vi "cupFinderv5.vi"(11 "image\n in":T1(plugin-control)) -> (0 "WORK FOR GODS SAKE 2":T1(plugin-control), 1 "X-Out":dbl, 2 "CupPosition":T1(plugin-control), 3 "Refnum out":T1(plugin-control), 4 "Y-Out":dbl, 5 "ImgToCrop":T1(plugin-control))   [LabVIEW 2017]
uses:
  <vilib>/vision/NI_Vision_Development_Module.lvlib
panel:
  out "ROI Descriptor":T2 {"Contours"."Type" items=["No Selection", "Point", "Line", "Rectangle", "Oval", "Polygon", "Freehand Region", "Annulus", "Unused2", "Unused3", "Broken Line", "Freehand Line", "Rotated Rectangle"]}
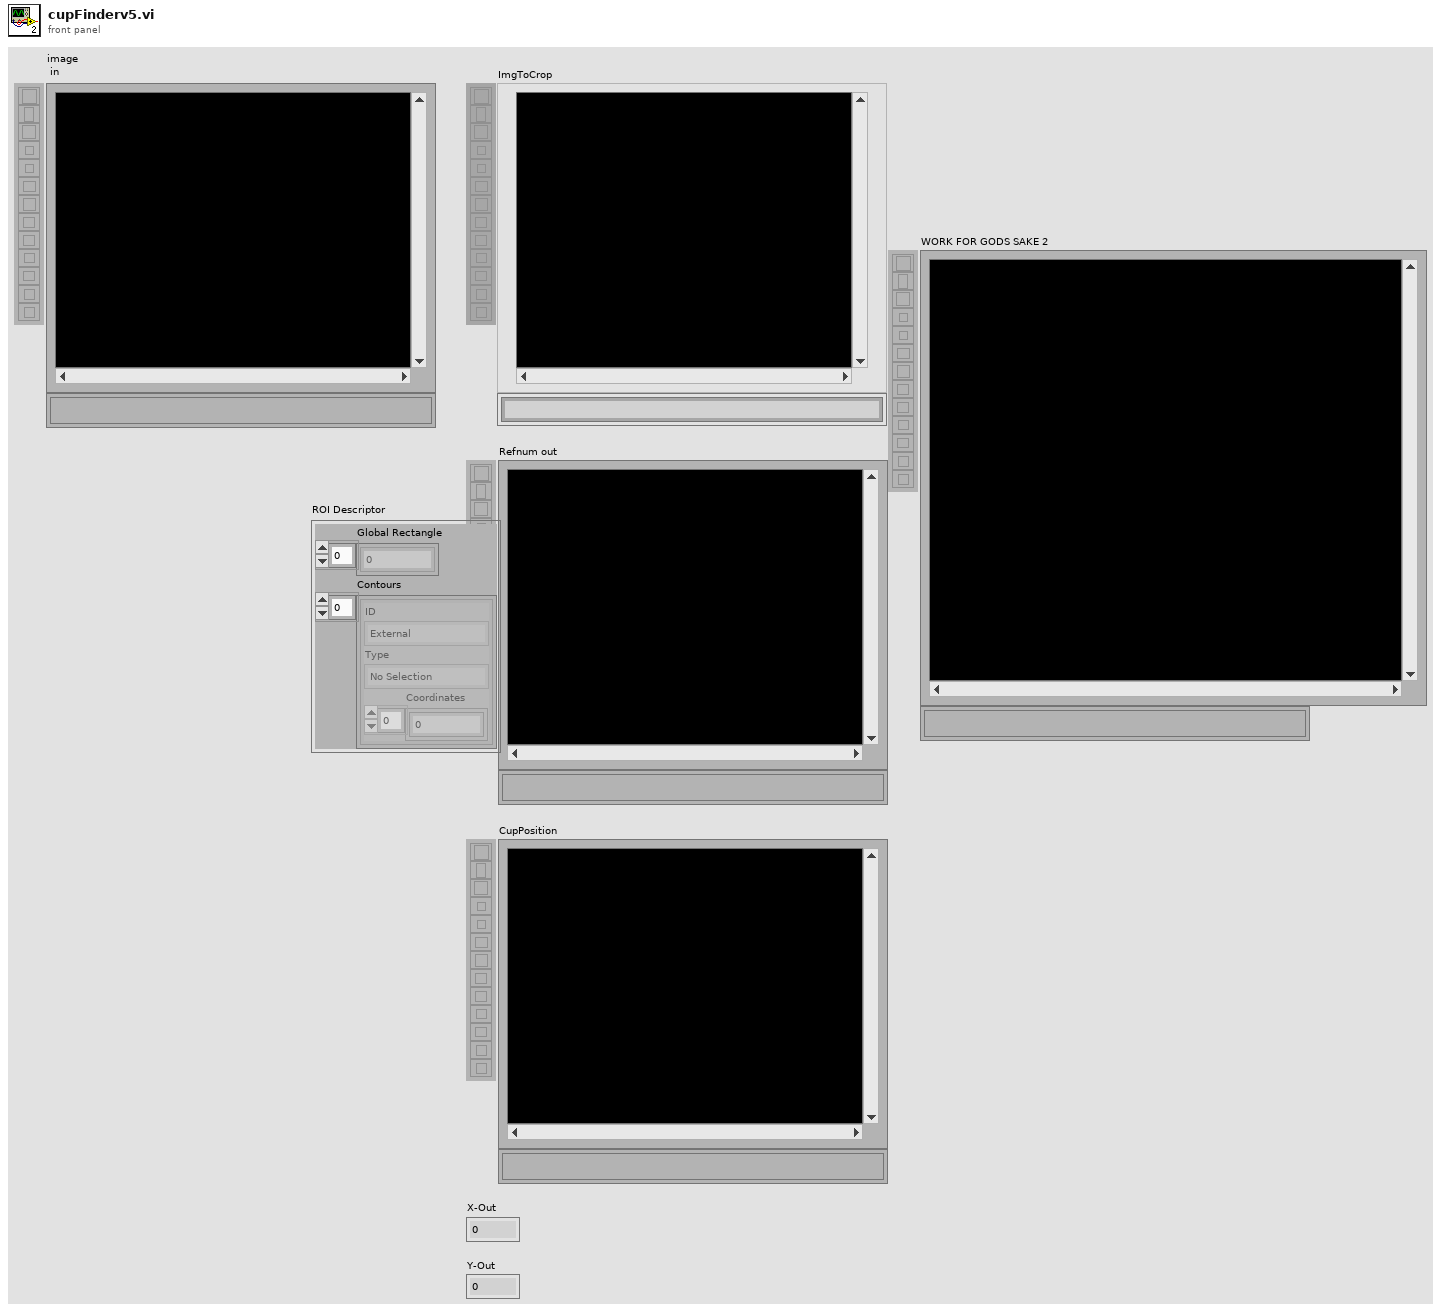
[diagram p1: front panel]
types:
  T1 = typedef "IMAQ Image.ctl" = refnum<image>
  T2 = cluster{"Global Rectangle":i32[], "Contours":cluster{"ID":enum32{"External", "Internal"}, "Type":u32, "Coordinates":i32[]}[]}
  T3 = typedef "Image Type" = u32
  T4 = cluster{"Position":cluster{"x":sgl, "y":sgl}, "Angle":sgl, "Scale":sgl, "Score":sgl, "Bounding Box":cluster{"x":sgl, "y":sgl}[]}[]
  T5 = typedef "IMAQ Rectangle" = cluster{"Left":i32, "Top":i32, "Right":i32, "Bottom":i32, "Rotation":dbl}
  T6 = typedef "ROI Descriptor" = cluster{"Global Rectangle":i32[], "Contours":cluster{"ID":enum32{"External", "Internal"}, "Type":u32, "Coordinates":i32[]}[]}
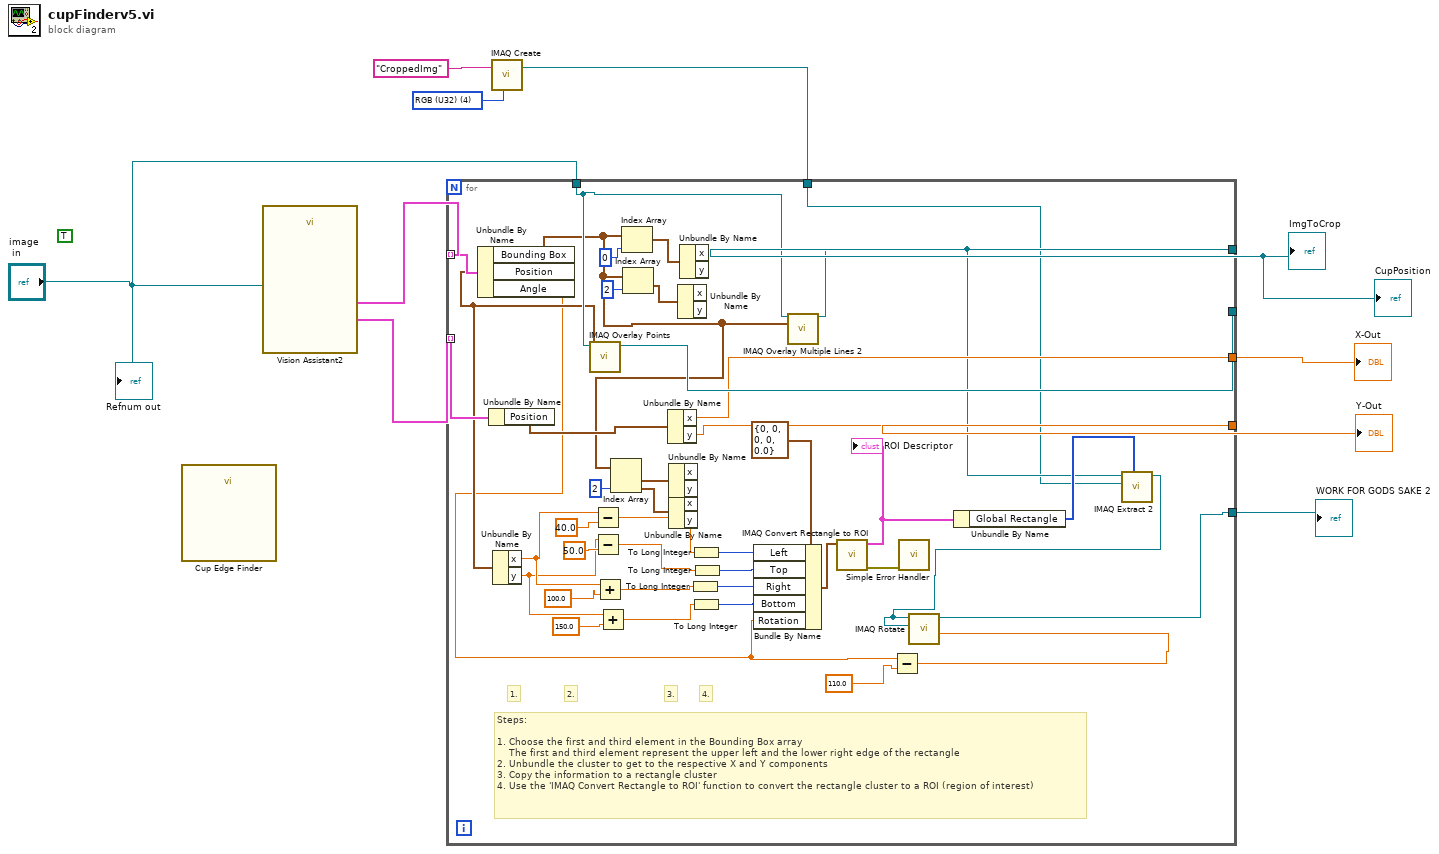
[diagram p0: block diagram]
diagram:
  w9 = T3 4 items=["Grayscale (U8)", "Grayscale (I16)", "Grayscale (SGL)", "Complex (CSG)", "RGB (U32)", "HSL (U32)", "RGB (U64)", "Grayscale (U16)"] ("Image Type")
  (unwired) TRUE
  n1 = call "Cup Edge Finder"() -> ()  [unwired: 25 in, 3 out]
  n2 = call "Vision Assistant2"("Image In"="image\n in") -> ("Calibrated Matches (Pattern Matching 5)"=w2:T4, "Matches (Pattern Matching 5)"=w3:T4)  [unwired: 23 in, 2 out]
  n3 = call "IMAQ Create"("Image Name"="CroppedImg", "Image Type"=w9) -> ("New Image"=w10:T1)  [unwired: 3 in, 1 out]
  n4 = for {
    tunnel: [w28] -> w1
    tunnel: [w52] -> _
    tunnel: [w50] -> w6
    tunnel: [w49] -> w7
    tunnel: "image\n in" -> [w42]
    tunnel: w3 -> [w47] mode=indexing
    tunnel: w2 -> [w48] mode=indexing
    tunnel: w10 -> [w27]
    tunnel: [w14] -> w5
    # "1."
    # "2."
    # "3."
    # "4."
    # "Steps:\n\n1. Choose the first and third element in the Bounding Box array\n    The first and third element represent the upper left and the lower right edge of the rectangle\n2. Unbundle the cluster to get to the respective X and Y components\n3. Copy the information to a rectangle cluster\n4. Use the 'IMAQ Convert Rectangle to ROI' function to convert the rectangle cluster to a ROI (region of interest)"
    n5 = Unbundle By Name(w47) -> ("Bounding Box"=w29:cluster{"x":sgl, "y":sgl}[], "Position"=w26:cluster{"x":sgl, "y":sgl}, "Angle"=w12:sgl)
    n6 = Unbundle By Name(w48) -> ("Position"=w51:cluster{"x":sgl, "y":sgl})
    n7 = Unbundle By Name(w26) -> ("x"=w21:sgl, "y"=w18:sgl)
    n8 = call "IMAQ Overlay Points"("Point"=w26, "Image"=w42) -> ("Image Out"=w52:T1)  [unwired: 8 in, 1 out]
    n9 = Subtract(x=w21, y=sgl 40.0) -> (x-y=w24:sgl)
    n10 = Subtract(x=w18, y=sgl 50.0) -> (x-y=w22:sgl)
    n11 = Add(x=w21, y=sgl 100.0) -> (x+y=w19:sgl)
    n12 = Add(x=w18, y=sgl 150.0) -> (x+y=w16:sgl)
    n13 = Index Array(array=w29, index #2=2 ("index")) -> (element #1=w40:cluster{"x":sgl, "y":sgl}, element #2=w39:cluster{"x":sgl, "y":sgl})  [unwired: 1 in]
    n14 = Index Array(array=w29, index=0) -> (element=w45:cluster{"x":sgl, "y":sgl})
    n15 = Index Array(array=w29, index=2) -> (element=w43:cluster{"x":sgl, "y":sgl})
    n16 = Unbundle By Name(w51) -> ("x"=w50:sgl, "y"=w49:sgl)
    n17 = Unbundle By Name(w40) -> ()  [unwired: 2 out]
    n18 = Unbundle By Name(w39) -> ()  [unwired: 2 out]
    n19 = Unbundle By Name(w43) -> ()  [unwired: 2 out]
    n20 = Unbundle By Name(w45) -> ()  [unwired: 2 out]
    n21 = To Long Integer(number=w19) -> (32bit integer=w34:i32)
    n22 = To Long Integer(number=w24) -> (32bit integer=w36:i32)
    n23 = To Long Integer(number=w16) -> (32bit integer=w33:i32)
    n24 = To Long Integer(number=w22) -> (32bit integer=w35:i32)
    n25 = Bundle By Name(cluster=T5 {"Left"=0, "Top"=0, "Right"=0, "Bottom"=0, "Rotation"=0.0} ("Rectangle"), "Left"=w36, "Top"=w35, "Right"=w34, "Bottom"=w33, "Rotation"=w12) -> (w38:T5)
    n26 = call "IMAQ Overlay Multiple Lines 2"("Image"=w42, "Line End Points"=w29) -> ("Image Out"=w28:T1)  [unwired: 12 in, 1 out]
    n27 = call "IMAQ Convert Rectangle to ROI"("Rectangle"=w38) -> ("error out"=w32:errorcluster, "ROI Descriptor"=w31:T6)  [unwired: 8 in]
    "ROI Descriptor" <- w31
    n28 = Subtract(x=w12, y=sgl 110.0) -> (x-y=w11:sgl)
    n29 = call <vilib>:"Simple Error Handler.vi"("error in (no error)"=w32) -> ()  [unwired: 4 in, 5 out]
    n30 = Unbundle By Name(w31) -> ("Global Rectangle"=w30:i32[])
    n31 = call "IMAQ Extract 2"("Optional Rectangle"=w30, "Image Dst"=w27, "Image Src"=w28) -> ("Image Dst Out"=w15:T1)  [unwired: 7 in, 1 out]
    n32 = call "IMAQ Rotate"("Angle (degrees)"=w11, "Image Dst"=w15, "Image Src"=w15) -> ("Image Dst Out"=w14:T1)  [unwired: 7 in, 1 out]
  }
  "ImgToCrop" <- w1
  "CupPosition" <- w1
  "X-Out" <- w6
  "Y-Out" <- w7
  "WORK FOR GODS SAKE 2" <- w5
  "Refnum out" <- "image\n in"
